vi "Vacuum_pressure_check.vi"(3 "error in":errorcluster, 4 "Step Number in":i32, 5 "Data in":T1) -> (0 "error out":errorcluster, 1 "Step Number out":i32, 2 "Data out":T1)   [LabVIEW 2015, in "Steps.lvlib"]
uses:
  Steps.lvlib
  Type_Defs/Data.ctl
  Type_Defs/Diagnostics.ctl
  Type_Defs/Systems.ctl
panel:
  in  "Step Back":bool
  in  "Continue":bool
  out "Vacuum Pressure":dbl
  # "Options"
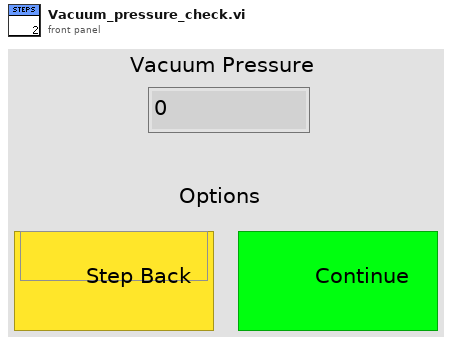
[diagram p1: front panel]
types:
  T1 = typedef "Data.ctl" = cluster{"User Name":string, "Experiment Number":i32, "Start Time":timestamp, "Data":dbl[], "Step Number":i32, "Step Instructions":string, "Diagnostics":T2, "Experiment Purpose":string, "Experiment State":enum16{"Off", "Setting Up", "Ready", "In Progress", "Shutting Down"}, "Systems":T3, "Current Pressure":dbl, "Fieldpoints":cluster{"System Boolean Fieldpoints":cluster{"Compressed Air":refnum<k21>, "T-20kV Power Switch":refnum<k21>, "T-Rectifier":refnum<k21>, "Engage Interlock":refnum<k21>, "Ventilator":refnum<k21>, "Magnetron":refnum<k21>, "H-20kV Power Switch":refnum<k21>, "H-Rectifier":refnum<k21>, "Main Water Pump":refnum<k21>, "WEGA Water Pump":refnum<k21>, "Gas Inlet Valves":refnum<k21>}, "Step Fieldpoints":cluster{"Exhaust Ventillator":refnum<k21>, "Compressed Air":refnum<k21>}}, "Pressure History":cluster{"Seconds into Experiement":i32[], "Pressure Data":dbl[]}}
  T2 = typedef "Diagnostics.ctl" = cluster{"Langmuir Probe":bool, "Rogowski 1":bool, "Rogowski 2":bool, "Rogowski 3":bool, "B-dot 1":bool, "B-dot 2":bool}
  T3 = typedef "Systems.ctl" = cluster{"Compressed Air":bool, "T-20kV Power Switch":bool, "T-Rectifier":bool, "Engage Interlock":bool, "Ventilator":bool, "Magnetron":bool, "H-20kV Power Switch":bool, "H-Rectifier":bool, "Main Water Pump":bool, "WEGA Water Pump":bool, "Gas Inlet Valves":bool}
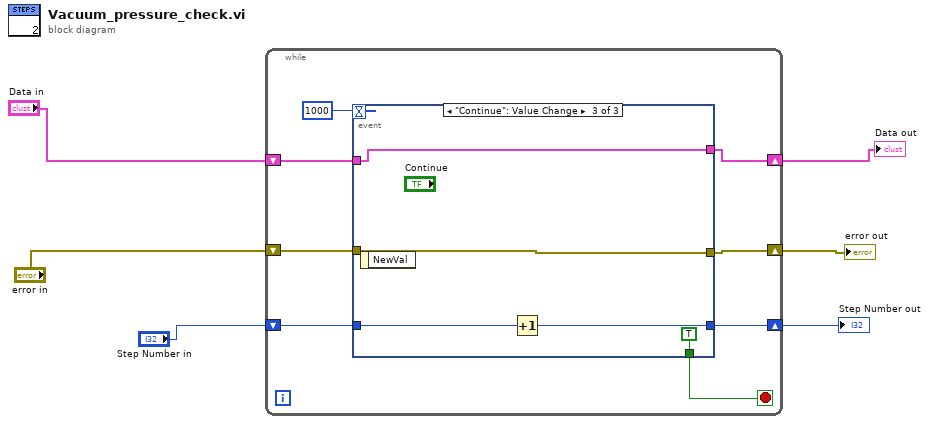
[diagram p0: block diagram]
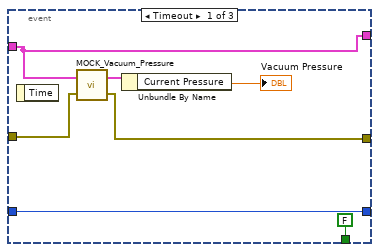
[diagram p2: hidden frame]
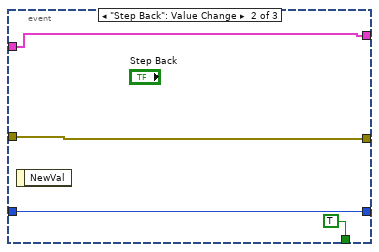
[diagram p3: hidden frame]
diagram:
  n1 = while {
    shift-right: [w13] -> w6
    shift-left: "error in" -> [w12]
    shift-right: [w10] -> w3
    shift-left: "Data in" -> [w11]
    shift-right: [w8] -> w1
    shift-left: "Step Number in" -> [w9]
    stop <- w7 stop-if-true
    n2 = event shown="[2] \"Continue\": Value Change" {
      selector: _ -> [_ _ _]
      dyn-events: _ -> [_ _ _]
      timeout: u32 1000 ("milliseconds to wait") -> [_ _ _]
      tunnel: [w19 w24 w30] -> w13
      tunnel: w12 -> [w18 w24 w30]
      tunnel: w11 -> [w17 w25 w29]
      tunnel: [w17 w25 w29] -> w10
      tunnel: w9 -> [w16 w23 w27]
      tunnel: [w16 w23 w28] -> w8
      tunnel: [FALSE TRUE TRUE] -> w7
      event Timeout {
        n3 = event-data() -> ()  [unwired: 1 in, 1 out]
        n4 = call "MOCK_Vacuum_Pressure.vi"("error constant"=w18, "Data in"=w17) -> ("error constant 2"=w19:errorcluster, "Data out"=w20:T1)
        n5 = Unbundle By Name(w20) -> ("Current Pressure"=→"Vacuum Pressure":dbl)
      }
      event "Step Back": Value Change {
        n6 = event-data() -> ()  [unwired: 1 in, 1 out]
      }
      event "Continue": Value Change {
        n7 = event-data() -> ()  [unwired: 1 in, 1 out]
        n8 = Increment(x=w27) -> (x+1=w28:i32)
      }
    }
  }
  "error out" <- w6
  "Data out" <- w3
  "Step Number out" <- w1
